vi "RFmx_MeasTest_Config_InLoop.vi"(7 "Meas_Type":string[](array[string]), 8 "error in (no error)":errorcluster, 11 "Instrument Handle in":refnum<k21>="VST") -> (0 "error out":errorcluster, 3 "Instrument Handle out":refnum<k21>="VST")   [LabVIEW 2014]
uses:
  <vilib>/RFmx/RFInstr/mx/RFmxInstr.llb/RFmxInstr Build Signal String.vi
panel:
  in  "SFDR_Span(Hz)":dbl=20000000.0 format="%#_6p"
  in  "Acq_Time":dbl=0.01 format="%#_6p"
  in  "OBW_Percent":dbl=95.0 format="%#_6p"
  in  "Offset_IBW":dbl[](array[numeric])=[3840000.0, 3840000.0, 3840000.0] format="%#_6p"
  in  "Offset_Freq":dbl[](array[numeric])=[5000000.0, 10000000.0, 12500000.0] format="%#_6p"
  in  "Ch_IBW":dbl=3840000.0 format="%#_6p"
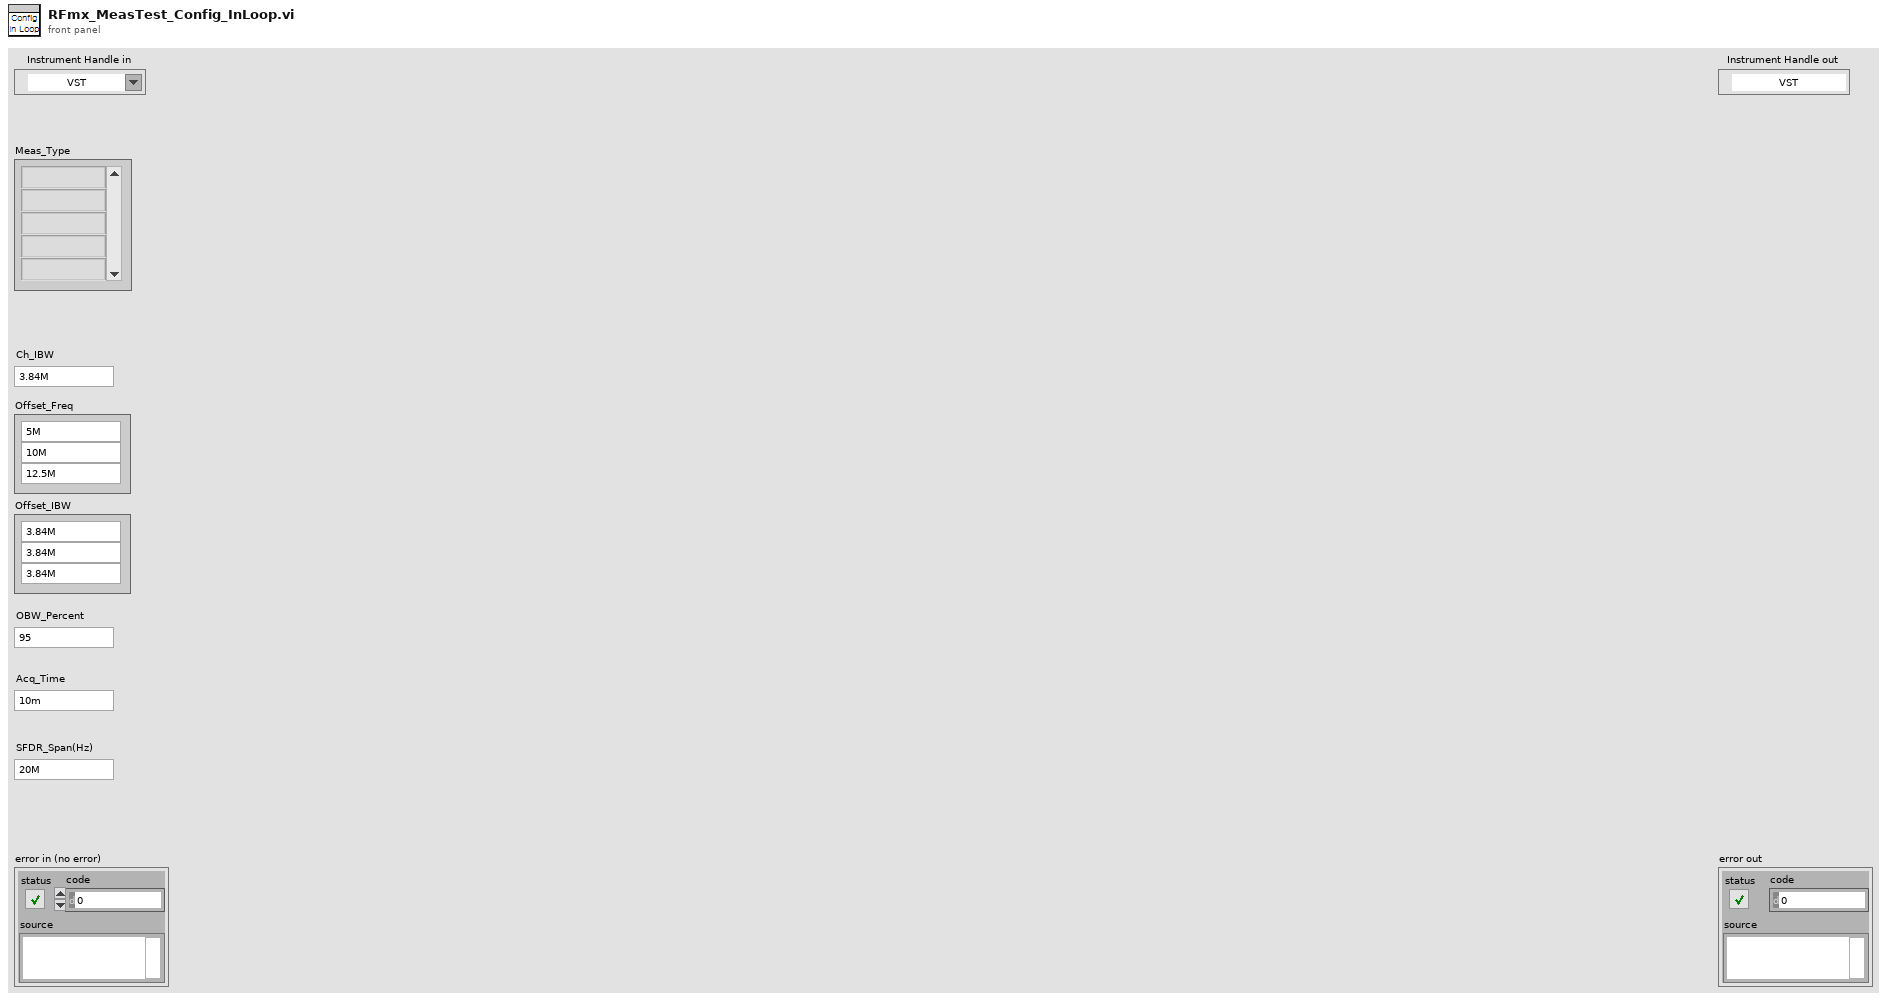
[diagram p1: front panel]
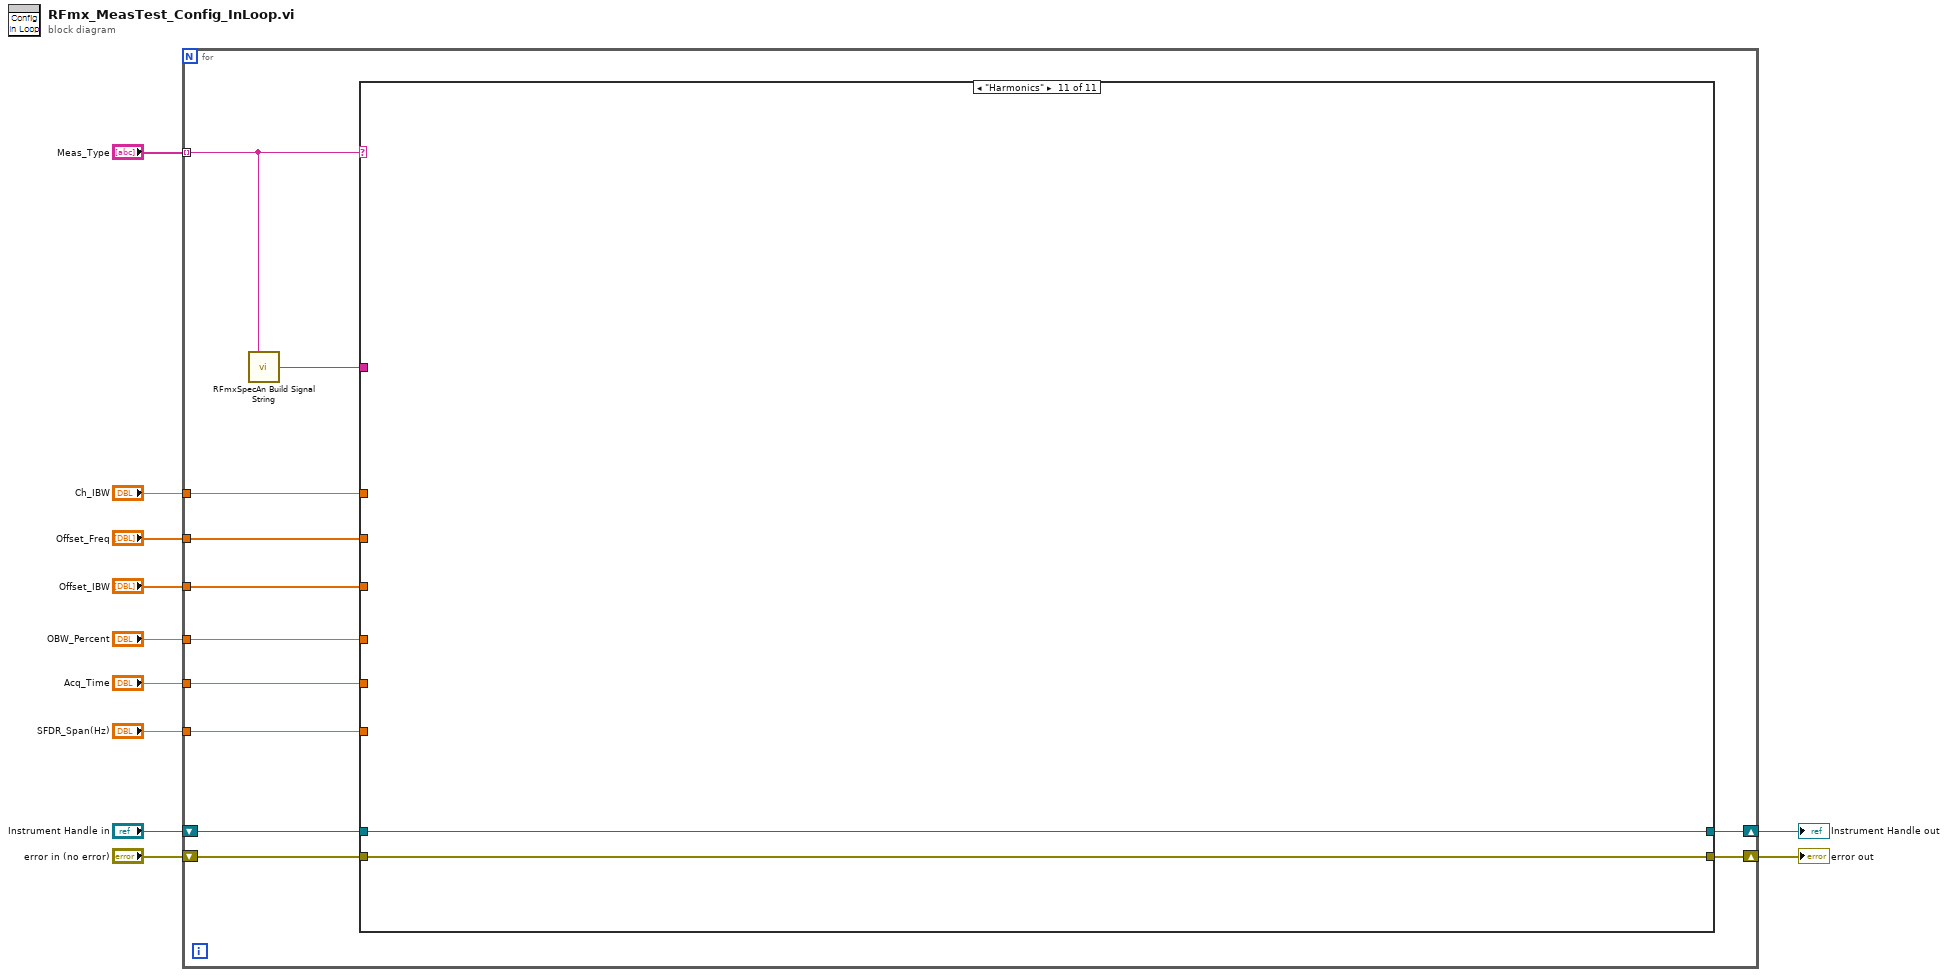
[diagram p0: block diagram]
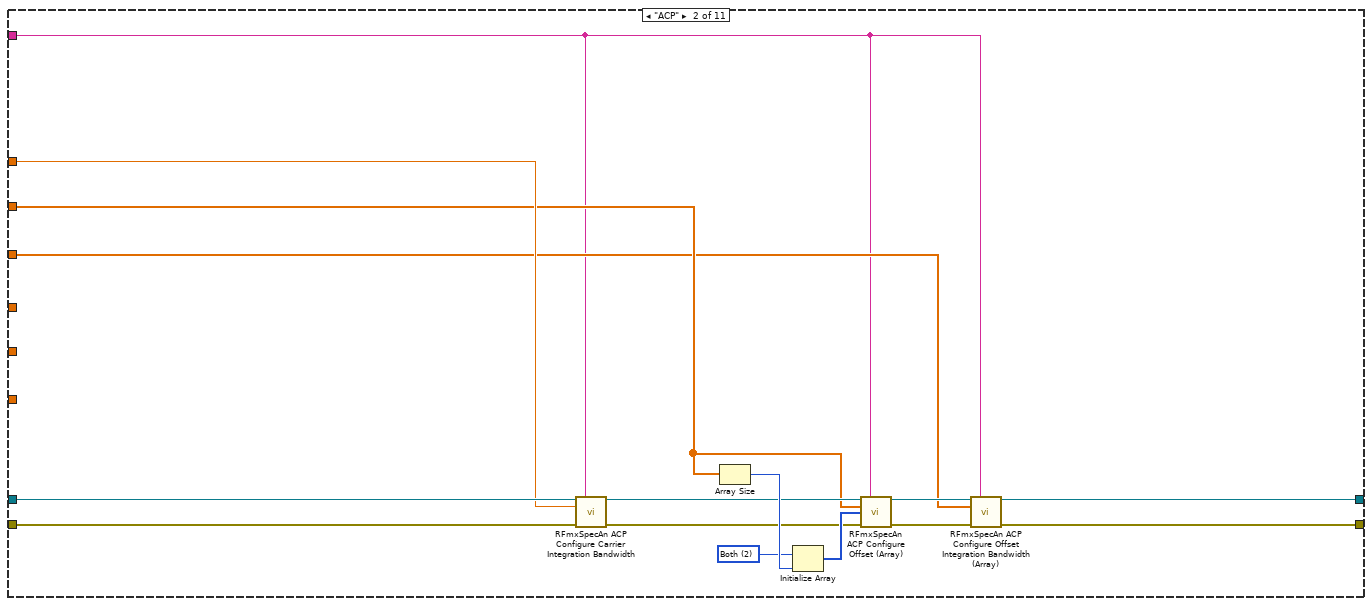
[diagram p3: hidden frame]
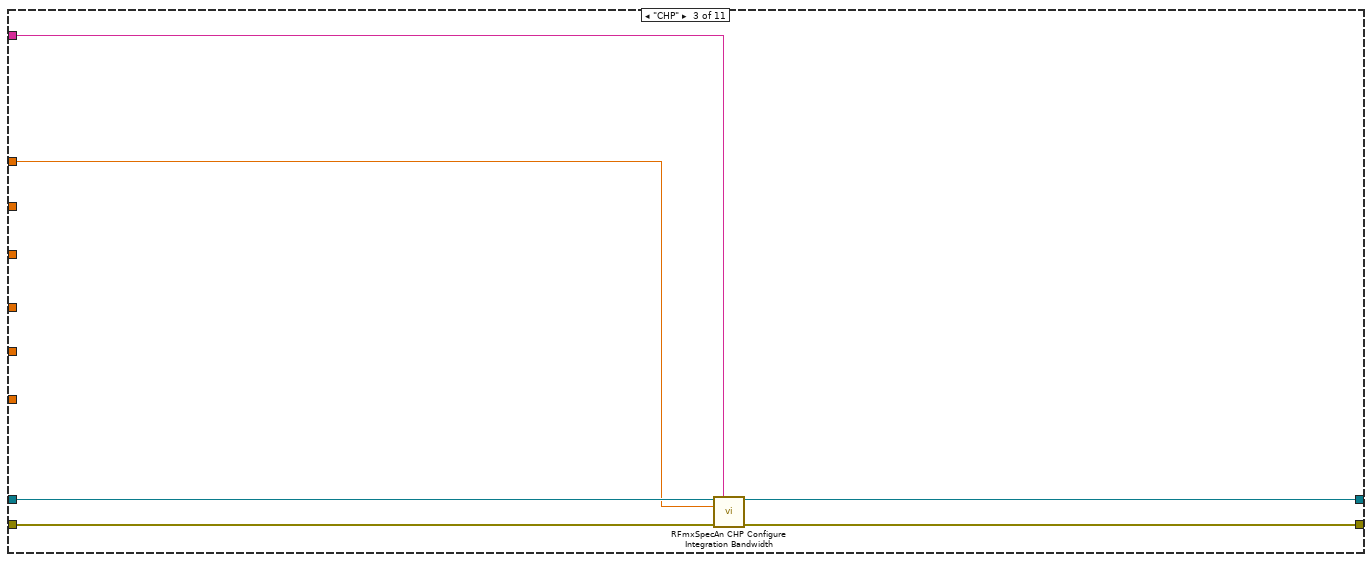
[diagram p4: hidden frame]
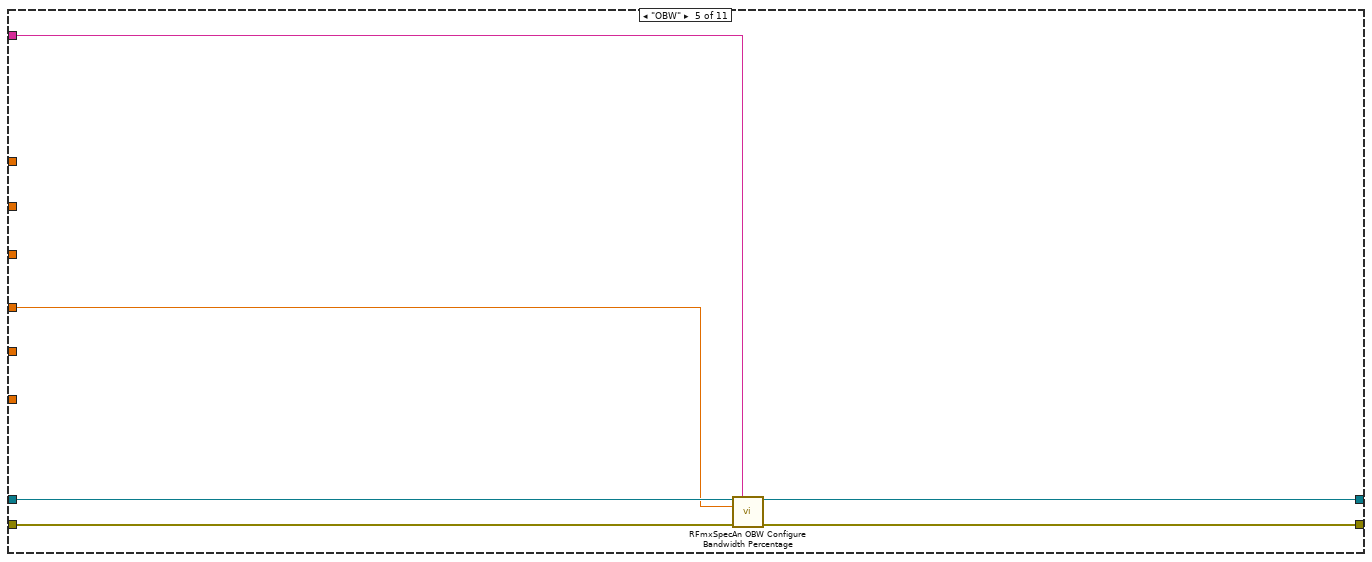
[diagram p6: hidden frame]
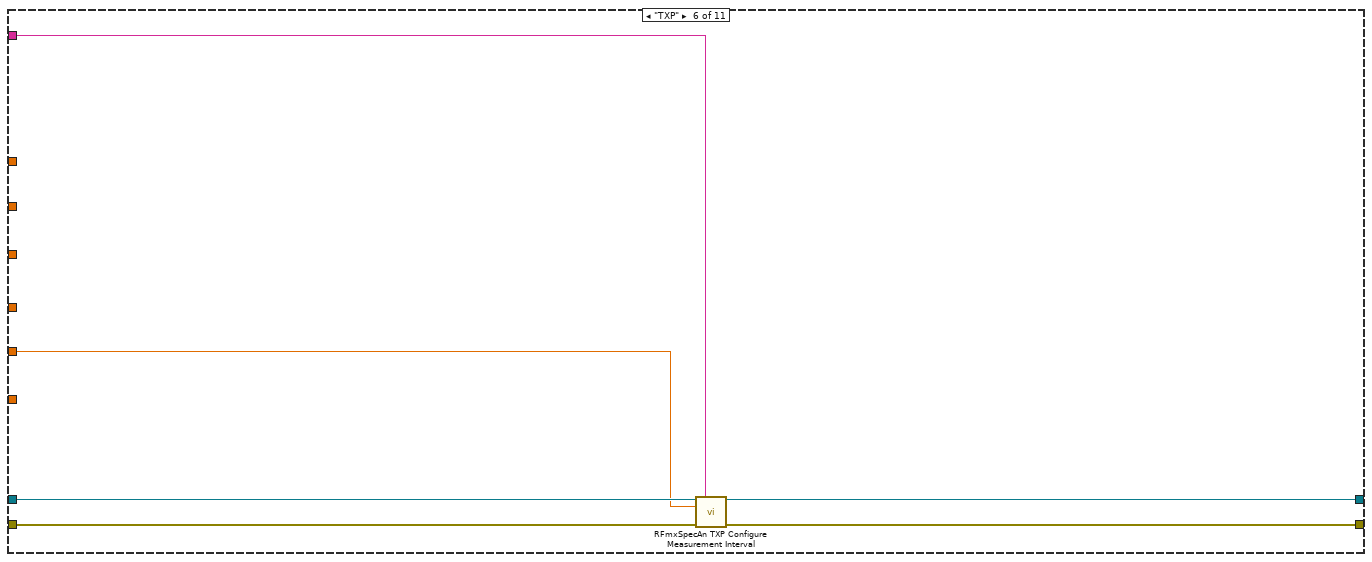
[diagram p7: hidden frame]
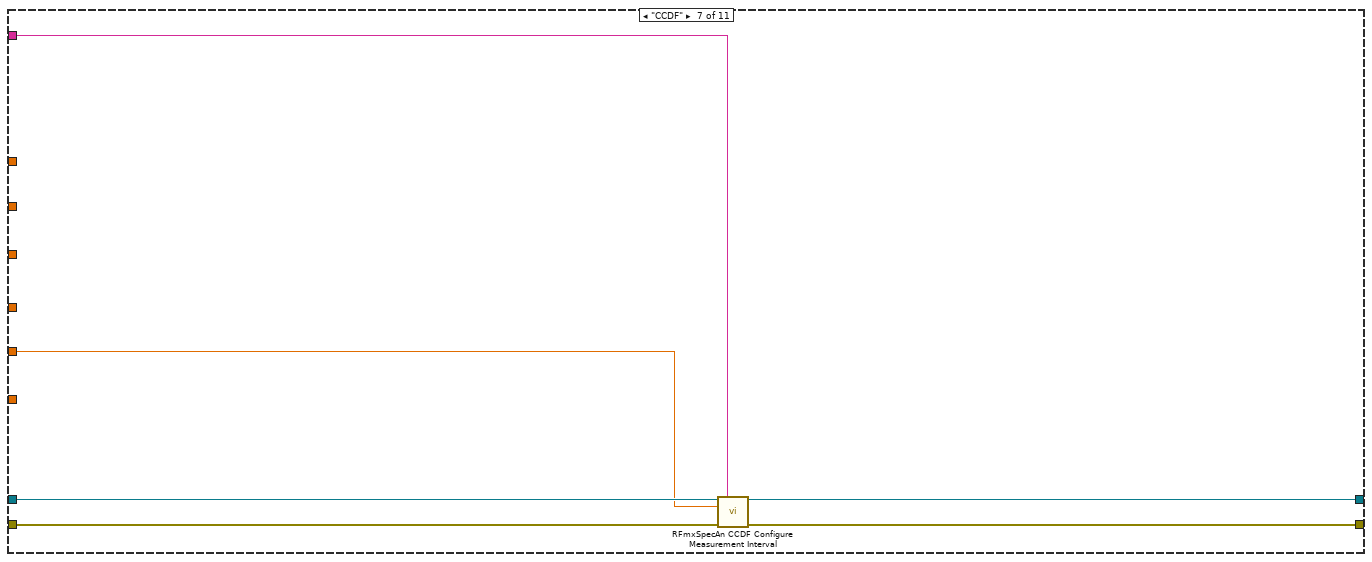
[diagram p8: hidden frame]
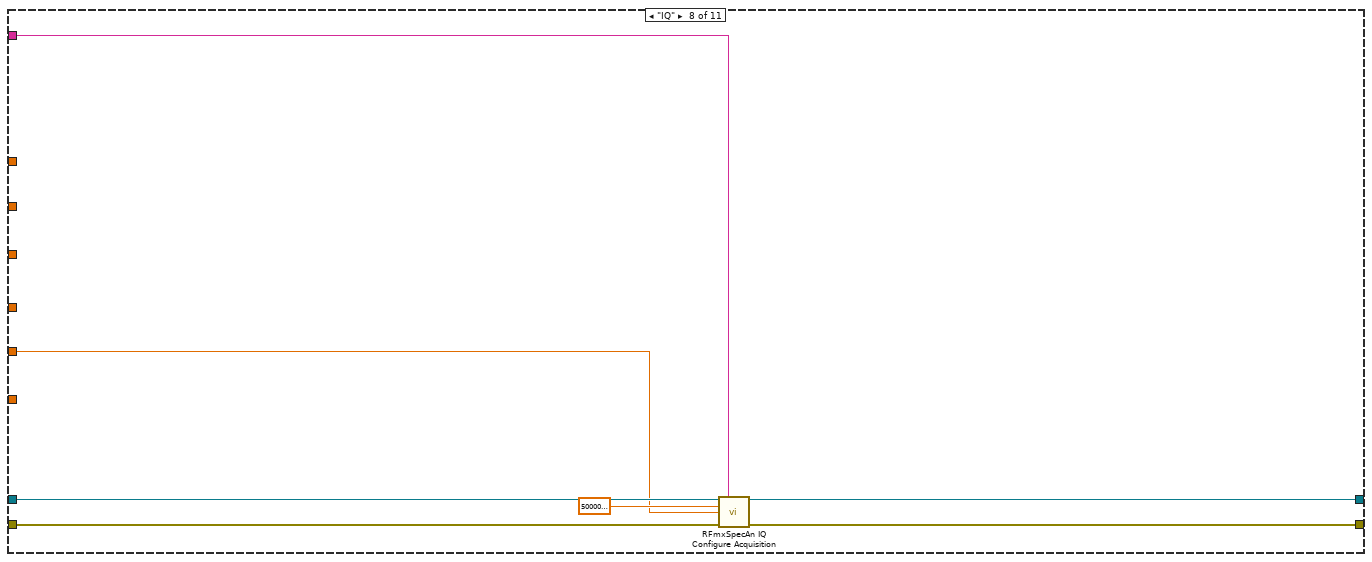
[diagram p9: hidden frame]
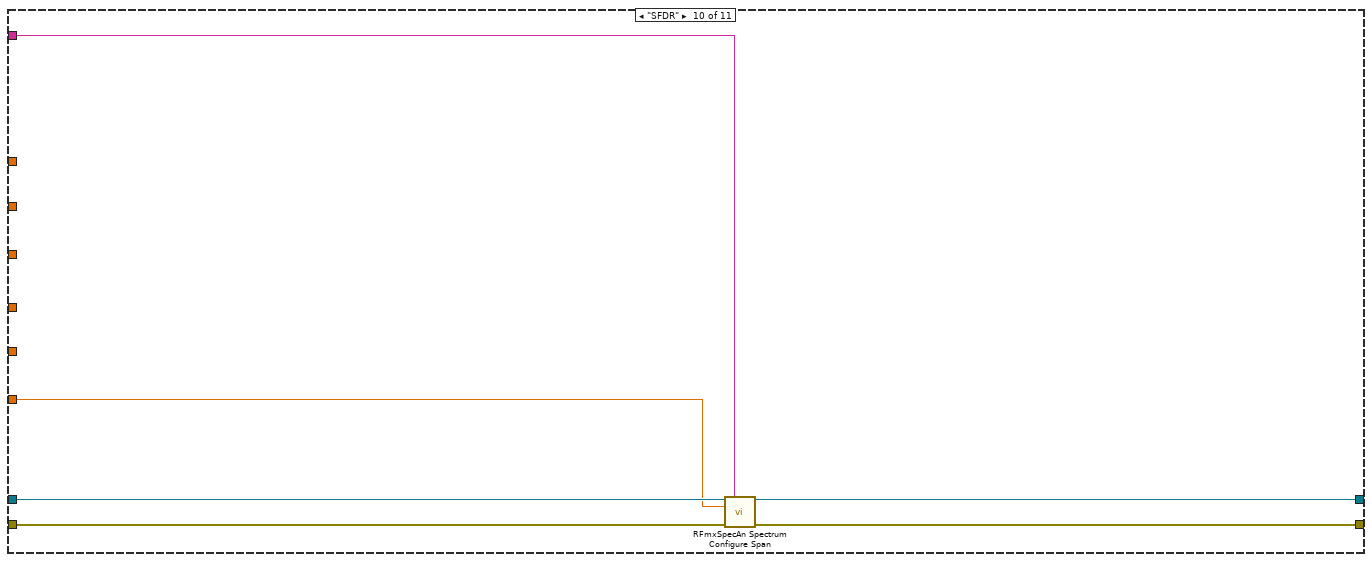
[diagram p11: hidden frame]
diagram:
  n1 = for {
    tunnel: "Ch_IBW" -> [w19]
    tunnel: "Offset_Freq" -> [w18]
    tunnel: "Offset_IBW" -> [w17]
    tunnel: "OBW_Percent" -> [w16]
    tunnel: "Acq_Time" -> [w15]
    tunnel: "SFDR_Span(Hz)" -> [w14]
    shift-right: [w20] -> w8
    shift-left: "Instrument Handle in" -> [w23]
    shift-right: [w21] -> w9
    shift-left: "error in (no error)" -> [w22]
    tunnel: "Meas_Type" -> [w13] mode=indexing
    n2 = call <vilib>:"RFmxSpecAn Build Signal String.vi"("Signal Name"=w13) -> ("Selector String"=w12:string)  [unwired: 14 in]
    n3 = case shown="\"Harmonics\"" w13 {
      tunnel: w23 -> [w25 w33 w46 w48 w54 w60 w66 w73 w75 w81 w83]
      tunnel: w22 -> [w24 w32 w45 w47 w53 w59 w65 w72 w74 w80 w82]
      tunnel: [w25 w31 w43 w48 w52 w58 w63 w71 w75 w79 w83] -> w20
      tunnel: [w24 w30 w42 w47 w51 w57 w62 w70 w74 w78 w82] -> w21
      tunnel: w19 -> [_ w29 w44 _ _ _ _ _ _ _ _]
      tunnel: w18 -> [_ w28 _ _ _ _ _ _ _ _ _]
      tunnel: w17 -> [_ w27 _ _ _ _ _ _ _ _ _]
      tunnel: w16 -> [_ _ _ _ w50 _ _ _ _ _ _]
      tunnel: w15 -> [_ _ _ _ _ w56 w64 w68 _ _ _]
      tunnel: w14 -> [_ _ _ _ _ _ _ _ _ w77 _]
      tunnel: w12 -> [_ w26 w41 _ w49 w55 w61 w67 _ w76 _]
      frame "Spectrum", Default {
      }
      frame "ACP" {
        w38 = 2 items=["Neg", "Pos", "Both"] ("Offset Frequency Sideband")
        n4 = call <vilib>:"RFmxSpecAn ACP Configure Carrier Integration Bandwidth.vi"("Instrument Handle In"=w33, "Selector String"=w26, "Integration Bandwidth (Hz)"=w29, "error in (no error)"=w32) -> ("Instrument Handle Out"=w35:refnum<k21>, "error out"=w34:errorcluster)  [unwired: 10 in]
        n5 = Array Size(array=w28) -> (size(s)=w39:i32)
        n6 = Initialize Array(w38, w39) -> (w40:i32[])
        n7 = call <vilib>:"RFmxSpecAn ACP Configure Offset (Array).vi"("Instrument Handle In"=w35, "Selector String"=w26, "Offset Frequency (Hz)"=w28, "Offset Sideband"=w40, "error in (no error)"=w34) -> ("Instrument Handle Out"=w36:refnum<k21>, "error out"=w37:errorcluster)  [unwired: 9 in]
        n8 = call <vilib>:"RFmxSpecAn ACP Configure Offset Integration Bandwidth (Array).vi"("Instrument Handle In"=w36, "Selector String"=w26, "Integration Bandwidth (Hz)"=w27, "error in (no error)"=w37) -> ("Instrument Handle Out"=w31:refnum<k21>, "error out"=w30:errorcluster)  [unwired: 10 in]
      }
      frame "CHP" {
        n9 = call <vilib>:"RFmxSpecAn CHP Configure Integration Bandwidth.vi"("Instrument Handle In"=w46, "Selector String"=w41, "Integration Bandwidth (Hz)"=w44, "error in (no error)"=w45) -> ("Instrument Handle Out"=w43:refnum<k21>, "error out"=w42:errorcluster)  [unwired: 10 in]
      }
      frame "FCnt" {
      }
      frame "OBW" {
        n10 = call <vilib>:"RFmxSpecAn OBW Configure Bandwidth Percentage.vi"("Instrument Handle In"=w54, "Selector String"=w49, "Bandwidth Percentage (%)"=w50, "error in (no error)"=w53) -> ("Instrument Handle Out"=w52:refnum<k21>, "error out"=w51:errorcluster)  [unwired: 10 in]
      }
      frame "TXP" {
        n11 = call <vilib>:"RFmxSpecAn TXP Configure Measurement Interval.vi"("Instrument Handle In"=w60, "Selector String"=w55, "Measurement Interval (s)"=w56, "error in (no error)"=w59) -> ("Instrument Handle Out"=w58:refnum<k21>, "error out"=w57:errorcluster)  [unwired: 10 in]
      }
      frame "CCDF" {
        n12 = call <vilib>:"RFmxSpecAn CCDF Configure Measurement Interval.vi"("Instrument Handle In"=w66, "Selector String"=w61, "Measurement Interval (s)"=w64, "error in (no error)"=w65) -> ("Instrument Handle Out"=w63:refnum<k21>, "error out"=w62:errorcluster)  [unwired: 10 in]
      }
      frame "IQ" {
        n13 = call <vilib>:"RFmxSpecAn IQ Configure Acquisition.vi"("Instrument Handle In"=w73, "Selector String"=w67, "Sample Rate (S/s)"=50000000.0, "Acquisition Time (s)"=w68, "error in (no error)"=w72) -> ("Instrument Handle Out"=w71:refnum<k21>, "error out"=w70:errorcluster)  [unwired: 9 in]
      }
      frame "IMD" {
      }
      frame "SFDR" {
        n14 = call <vilib>:"RFmxSpecAn Spectrum Configure Span.vi"("Instrument Handle In"=w81, "Selector String"=w76, "Span (Hz)"=w77, "error in (no error)"=w80) -> ("Instrument Handle Out"=w79:refnum<k21>, "error out"=w78:errorcluster)  [unwired: 10 in]
      }
      frame "Harmonics" {
      }
    }
  }
  "Instrument Handle out" <- w8
  "error out" <- w9
